vi "Parse VI.vi"(8 "error in (no error)":errorcluster, 11 "VI Binary Data in":string) -> (0 "error out":errorcluster, 3 "Content out":T1)   [LabVIEW 2021, in "VI-Hacker.lvlib"]
uses:
  VI-Hacker.lvlib
  TypeDefs/Content.ctl
  TypeDefs/Block.ctl
  TypeDefs/RSRC_Header.ctl
  TypeDefs/RSRC_Info.ctl
  TypeDefs/RSRC_Id.ctl
  <vilib>/Utility/error.llb/Error Cluster From Error Code.vi
  <vilib>/ErrorRing/Error Ring.xnode
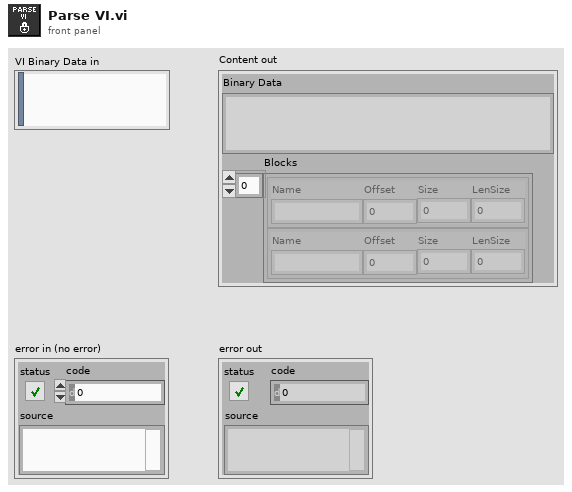
[diagram p1: front panel]
types:
  T1 = typedef "VI-Hacker.lvlib/Content.ctl" = cluster{"Binary Data":string, "Blocks":T2[]}
  T2 = typedef "VI-Hacker.lvlib/Block.ctl" = cluster{"Name":string, "Offset":i32, "Size":i32, "LenSize":i32}
  T3 = typedef "VI-Hacker.lvlib/RSRC_Info.ctl" = cluster{"Int1":i32, "Int2":i32, "Int3":i32, "DataOffset":i32, "Int4":i32}
  T4 = typedef "VI-Hacker.lvlib/RSRC_Header.ctl" = cluster{"RSRC\\r\\n\\xx\\xx":u64, "LVINLBVW":u64, "RSRCOffset":i32, "RSRCSize":i32, "DataOffset":i32, "DataSize":i32}
  T5 = typedef "VI-Hacker.lvlib/RSRC_Id.ctl" = cluster{"Name":u32, "Count":u32, "Offset":i32}
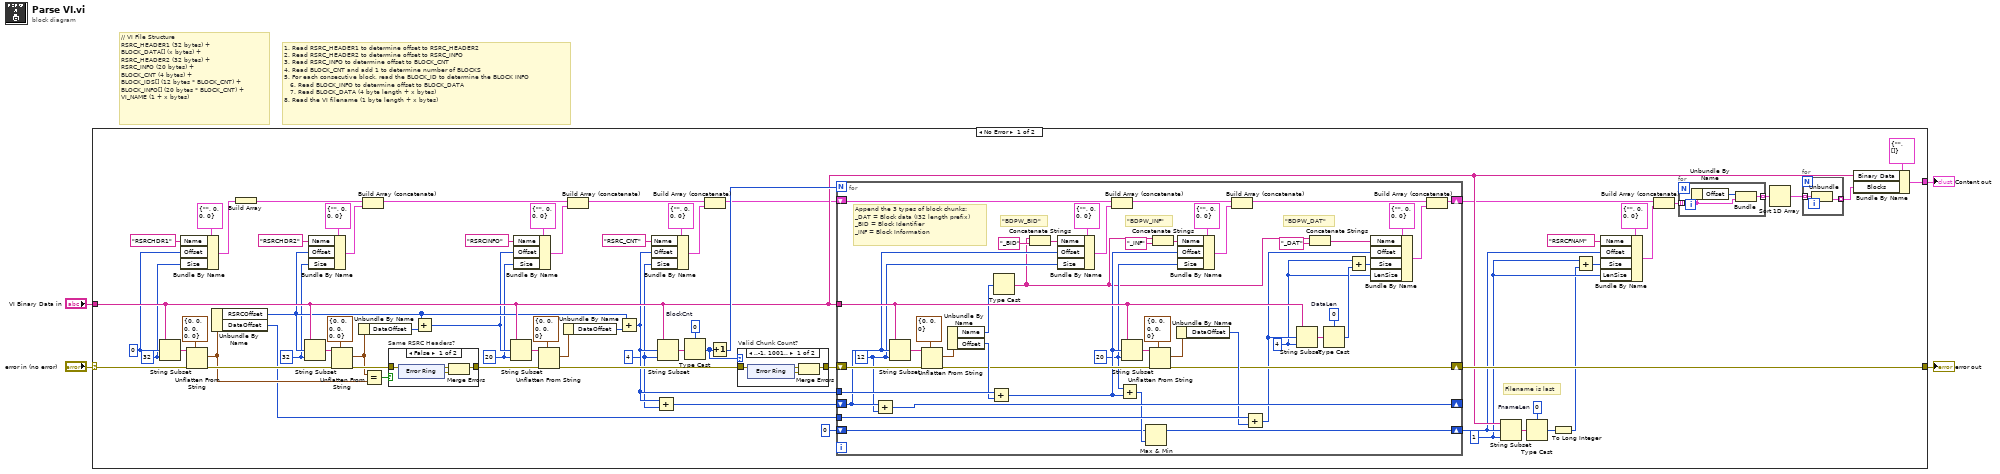
[diagram p0: block diagram]
diagram:
  # "1. Read RSRC_HEADER1 to determine offset to RSRC_HEADER2\n2. Read RSRC_HEADER2 to determine offset to RSRC_INFO\n3. Read RSRC_INFO to determine offset to BLOCK_CNT\n4. Read BLOCK_CNT and add 1 to determine number of BLOCKS\n5. For each consecutive block, read the BLOCK_ID to determine the BLOCK INFO\n   6. Read BLOCK_INFO to determine offset to BLOCK_DATA\n   7. Read BLOCK_DATA (4 byte length + x bytes)\n8. Read the VI filename (1 byte length + x bytes)"
  # "// VI File Structure\nRSRC_HEADER1 (32 bytes) + \nBLOCK_DATA[] (x bytes) +\nRSRC_HEADER2 (32 bytes) + \nRSRC_INFO (20 bytes) +\nBLOCK_CNT (4 bytes) + \nBLOCK_IDS[] (12 bytes * BLOCK_CNT) +\nBLOCK_INFO[] (20 bytes * BLOCK_CNT) +\nVI_NAME (1 + x bytes)"
  n1 = case shown="No Error" "error in (no error)" {
    selector: "error in (no error)" -> [w48 w140]
    tunnel: [w42 _] -> w4
    tunnel: [w52 w140] -> w3
    tunnel: "VI Binary Data in" -> [w43 _]
    frame No Error {
      w49 = u8 0  # FnameLen
      w16 = 1 ("length (rest)")
      w54 = 0  # BlockCnt
      w24 = 4 ("length (rest)")
      w31 = 20 ("length (rest)")
      w34 = 32 ("length (rest)")
      w39 = 32 ("length (rest)")
      w40 = 0 ("offset (0)")
      # "Filename is last"
      n2 = String Subset(string=w43, offset (0)=w40, length (rest)=w39) -> (substring=w71:string)
      n3 = Bundle By Name(cluster=T2 {"Name"="", "Offset"=0, "Size"=0, "LenSize"=0} ("Position"), "Name"="RSRCHDR1", "Offset"=w40, "Size"=w39) -> (w38:T2)
      n4 = Unflatten From String(type=T4 {"RSRC\\r\\n\\xx\\xx"=0, "LVINLBVW"=0, "RSRCOffset"=0, "RSRCSize"=0, "DataOffset"=0, "DataSize"=0} ("RSRC_HEADER"), binary string=w71, error in (no error)=w48) -> (value=w64:T4, error out=w72:errorcluster)  [unwired: 2 in, 1 out]
      n5 = Unbundle By Name(w64) -> ("RSRCOffset"=w35:i32, "DataOffset"=w57:i32)
      n6 = Build Array(w38) -> (w30:T2[])
      n7 = String Subset(string=w43, offset (0)=w35, length (rest)=w34) -> (substring=w70:string)
      n8 = Bundle By Name(cluster=T2 {"Name"="", "Offset"=0, "Size"=0, "LenSize"=0} ("Position"), "Name"="RSRCHDR2", "Offset"=w35, "Size"=w34) -> (w36:T2)
      n9 = Unflatten From String(type=T4 {"RSRC\\r\\n\\xx\\xx"=0, "LVINLBVW"=0, "RSRCOffset"=0, "RSRCSize"=0, "DataOffset"=0, "DataSize"=0} ("RSRC_HEADER"), binary string=w70, error in (no error)=w72) -> (value=w65:T4, error out=w67:errorcluster)  [unwired: 2 in, 1 out]
      n10 = Unbundle By Name(w65) -> ("DataOffset"=w69:i32)
      n11 = Build Array (concatenate)(w30, w36) -> (w29:T2[])
      n12 = Equal?(x=w65, y=w64) -> (x = y?=w68:bool)
      n13 = case "Same RSRC Headers?" shown="False" w68 {
        tunnel: w67 -> [w74 w80]
        tunnel: [w73 w80] -> w66
        frame False {
          n14 = xnode "Error Ring"() -> ("error out"=w75:errorcluster)
          n15 = Merge Errors(w74, w75) -> (w73:errorcluster)
        }
        frame True {
        }
      }
      n16 = Add(x=w35, y=w69) -> (x+y=w32:i32)
      n17 = String Subset(string=w43, offset (0)=w32, length (rest)=w31) -> (substring=w63:string)
      n18 = Bundle By Name(cluster=T2 {"Name"="", "Offset"=0, "Size"=0, "LenSize"=0} ("Position"), "Name"="RSRCINFO", "Offset"=w32, "Size"=w31) -> (w28:T2)
      n19 = Unflatten From String(type=T3 {"Int1"=0, "Int2"=0, "Int3"=0, "DataOffset"=0, "Int4"=0} ("RSRC_INFO"), binary string=w63, error in (no error)=w66) -> (value=w62:T3, error out=w56:errorcluster)  [unwired: 2 in, 1 out]
      n20 = Unbundle By Name(w62) -> ("DataOffset"=w61:i32)
      n21 = Build Array (concatenate)(w29, w28) -> (w23:T2[])
      n22 = Add(x=w35, y=w61) -> (x+y=w25:i32)
      n23 = Bundle By Name(cluster=T2 {"Name"="", "Offset"=0, "Size"=0, "LenSize"=0} ("Position"), "Name"="RSRC_CNT", "Offset"=w25, "Size"=w24) -> (w27:T2)
      n24 = Add(x=w25, y=w24) -> (x+y=w58:i32)
      n25 = String Subset(string=w43, offset (0)=w25, length (rest)=w24) -> (substring=w55:string)
      n26 = Type Cast(type=w54, x=w55) -> (*(type *) &x=w53:i32)
      n27 = Build Array (concatenate)(w23, w27) -> (w22:T2[])
      n28 = Increment(x=w53) -> (x+1=w59:i32)
      n29 = case "Valid Chunk Count?" shown="..-1, 1001.." w53 {
        tunnel: w56 -> [w128 w134]
        tunnel: [w127 w134] -> w60
        frame ..-1, 1001.. {
          n30 = xnode "Error Ring"() -> ("error out"=w129:errorcluster)
          n31 = Merge Errors(w128, w129) -> (w127:errorcluster)
        }
        frame 0..1000 {
        }
      }
      n32 = for {
        N: w59 -> [_]
        tunnel: w43 -> [w113]
        shift-right: [w124] -> _
        shift-left: w58 -> [w103]
        shift-right: [w112] -> w52
        shift-left: w60 -> [w126]
        tunnel: w25 -> [w122]
        tunnel: w57 -> [w118]
        shift-right: [w109] -> w17
        shift-left: 0 -> [w110]
        shift-right: [w93] -> w18
        shift-left: w22 -> [w104]
        w115 = 0  # DataLen
        w89 = 4 ("length (rest)")
        w97 = 20 ("length (rest)")
        w102 = 12 ("length (rest)")
        # "\"BDPW_DAT\""
        # "\"BDPW_INF\""
        # "\"BDPW_BID\""
        # "Append the 3 types of block chunks:\n_DAT = Block data (I32 length prefix)\n_BID = Block Identifier\n_INF = Block Information"
        n33 = Add(x=w103, y=w102) -> (x+y=w124:i32)
        n34 = String Subset(string=w113, offset (0)=w103, length (rest)=w102) -> (substring=w125:string)
        n35 = Unflatten From String(type=T5 {"Name"=0, "Count"=0, "Offset"=0} ("BLOCK_ID"), binary string=w125, error in (no error)=w126) -> (value=w123:T5, error out=w119:errorcluster)  [unwired: 2 in, 1 out]
        n36 = Unbundle By Name(w123) -> ("Name"=w88:u32, "Offset"=w121:i32)
        n37 = Add(x=w122, y=w121) -> (x+y=w98:i32)
        n38 = Type Cast(x=w88) -> (*(type *) &x=w84:string)  [unwired: 1 in]
        n39 = Concatenate Strings(w84, "_BID" ("string")) -> (w82:string)
        n40 = Bundle By Name(cluster=T2 {"Name"="", "Offset"=0, "Size"=0, "LenSize"=0} ("Position"), "Name"=w82, "Offset"=w103, "Size"=w102) -> (w105:T2)
        n41 = Build Array (concatenate)(w104, w105) -> (w99:T2[])
        n42 = Add(x=w97, y=w98) -> (x+y=w111:i32)
        n43 = String Subset(string=w113, offset (0)=w98, length (rest)=w97) -> (substring=w120:string)
        n44 = Max & Min(x=w110, y=w111) -> (max(x,y)=w109:i32)  [unwired: 1 out]
        n45 = Unflatten From String(type=T3 {"Int1"=0, "Int2"=0, "Int3"=0, "DataOffset"=0, "Int4"=0} ("RSRC_INFO"), binary string=w120, error in (no error)=w119) -> (value=w117:T3, error out=w112:errorcluster)  [unwired: 2 in, 1 out]
        n46 = Concatenate Strings(w84, "_INF" ("string")) -> (w81:string)
        n47 = Unbundle By Name(w117) -> ("DataOffset"=w116:i32)
        n48 = Bundle By Name(cluster=T2 {"Name"="", "Offset"=0, "Size"=0, "LenSize"=0} ("Position"), "Name"=w81, "Offset"=w98, "Size"=w97) -> (w101:T2)
        n49 = Build Array (concatenate)(w99, w101) -> (w94:T2[])
        n50 = Add(x=w118, y=w116) -> (x+y=w92:i32)
        n51 = String Subset(string=w113, offset (0)=w92, length (rest)=w89) -> (substring=w114:string)
        n52 = Concatenate Strings(w84, "_DAT" ("string")) -> (w83:string)
        n53 = Type Cast(type=w115, x=w114) -> (*(type *) &x=w91:i32)
        n54 = Add(x=w89, y=w91) -> (x+y=w90:i32)
        n55 = Bundle By Name(cluster=T2 {"Name"="", "Offset"=0, "Size"=0, "LenSize"=0} ("Position"), "Name"=w83, "Offset"=w92, "Size"=w90, "LenSize"=w89) -> (w95:T2)
        n56 = Build Array (concatenate)(w94, w95) -> (w93:T2[])
      }
      n57 = String Subset(string=w43, offset (0)=w17, length (rest)=w16) -> (substring=w50:string)
      n58 = Type Cast(type=w49, x=w50) -> (*(type *) &x=w14:u8)
      n59 = To Long Integer(number=w14) -> (32bit integer=w9:i32)
      n60 = Add(x=w16, y=w9) -> (x+y=w15:i32)
      n61 = Bundle By Name(cluster=T2 {"Name"="", "Offset"=0, "Size"=0, "LenSize"=0} ("Position"), "Name"="RSRCFNAM", "Offset"=w17, "Size"=w15, "LenSize"=w16) -> (w19:T2)
      n62 = Build Array (concatenate)(w18, w19) -> (w11:T2[])
      n63 = for {
        tunnel: w11 -> [w138] mode=indexing
        tunnel: [w137] -> w13 mode=indexing
        n64 = Unbundle By Name(w138) -> ("Offset"=w139:i32)
        n65 = Bundle("Offset"=w139, "Position"=w138) -> (w137:cluster{"Offset":i32, "Position":T2})  [unwired: 1 in]
      }
      n66 = Sort 1D Array(array=w13) -> (sorted array=w12:cluster{"Offset":i32, "Position":T2}[])
      n67 = for {
        tunnel: w12 -> [w136] mode=indexing
        tunnel: [w135] -> w10 mode=indexing
        n68 = Unbundle(w136) -> ("Position"=w135:T2)  [unwired: 1 out]
      }
      n69 = Bundle By Name(cluster=T1 {"Binary Data"="", "Blocks"=[]} ("Content out"), "Binary Data"=w43, "Blocks"=w10) -> (w42:T1)
    }
    frame Error {
    }
  }
  "error out" <- w3
  "Content out" <- w4
